vi "peak_detection.vi"(9 "spectrum cluster":T1, 10 "Minimum Peak Width":i32=5 min=3, 11 "Threshold Value":dbl=10.0) -> (1 "PeaksFound":i32)   [LabVIEW 2012]
uses:
  <vilib>/Analysis/baseanly.llb/Mean (DBL).vi
  <vilib>/measure/NI_MAPro.lvlib
  <vilib>/Analysis/NI_AALBase.lvlib
panel:
  in  "Stop":bool
  out "Amplitude":dbl[](array[numeric]) format="%.3p"
  out "Frequency":dbl[](array[numeric]) format="%.6p"
  out "Average Cor":cluster{"Array":dbl[], "magnitude":dbl[]}[](graph)
  # "Peak Detection"
  # "Detection Settings"
  # "Detected Peaks"
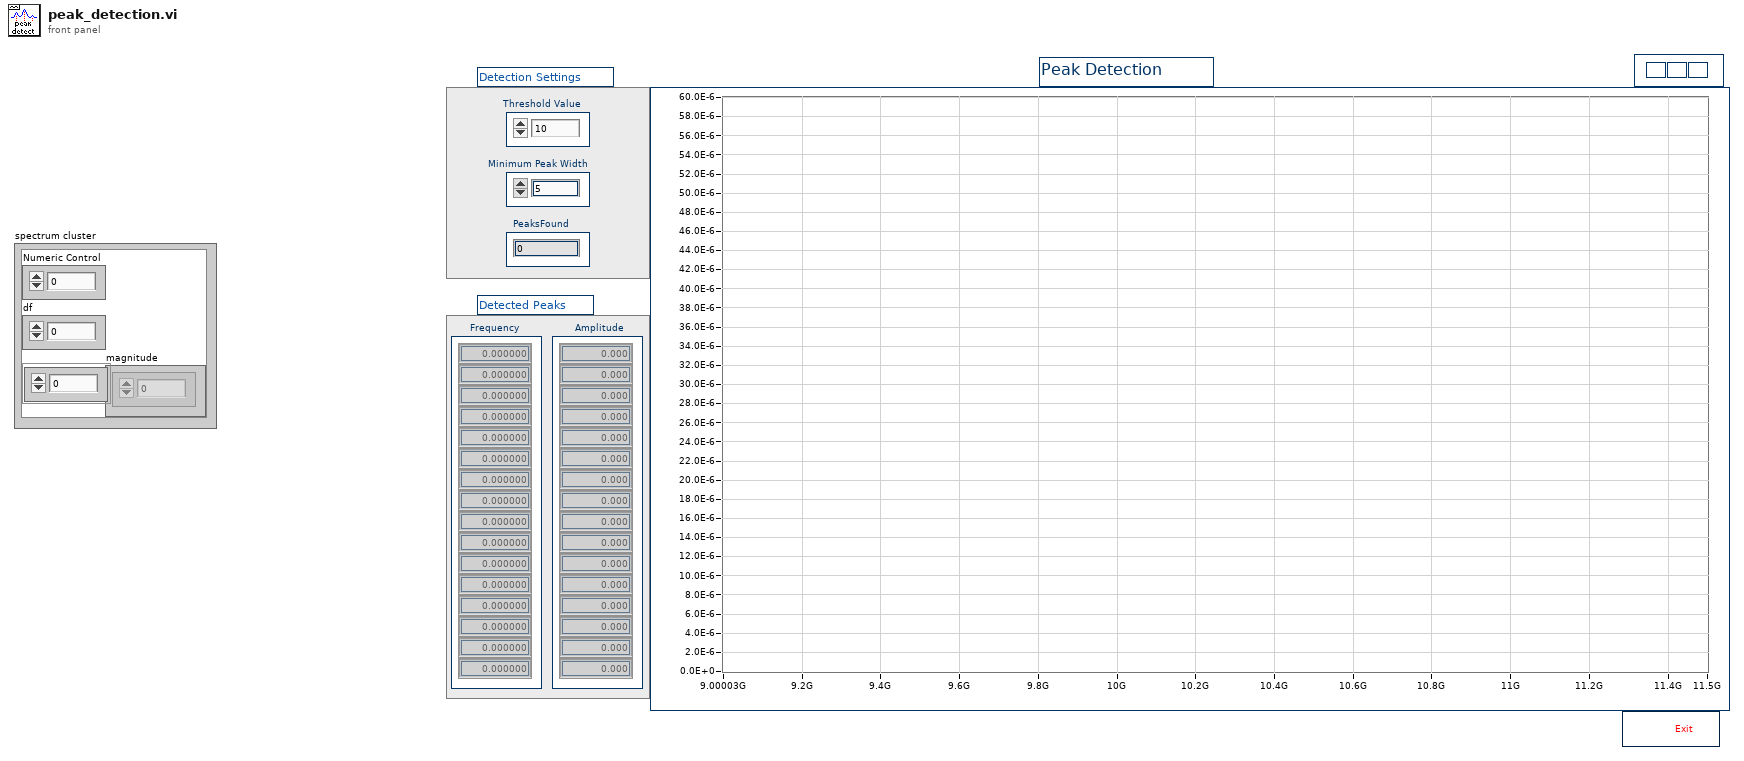
[diagram p1: front panel]
types:
  T1 = cluster{"Numeric Control":dbl, "df":dbl, "magnitude":dbl[]}
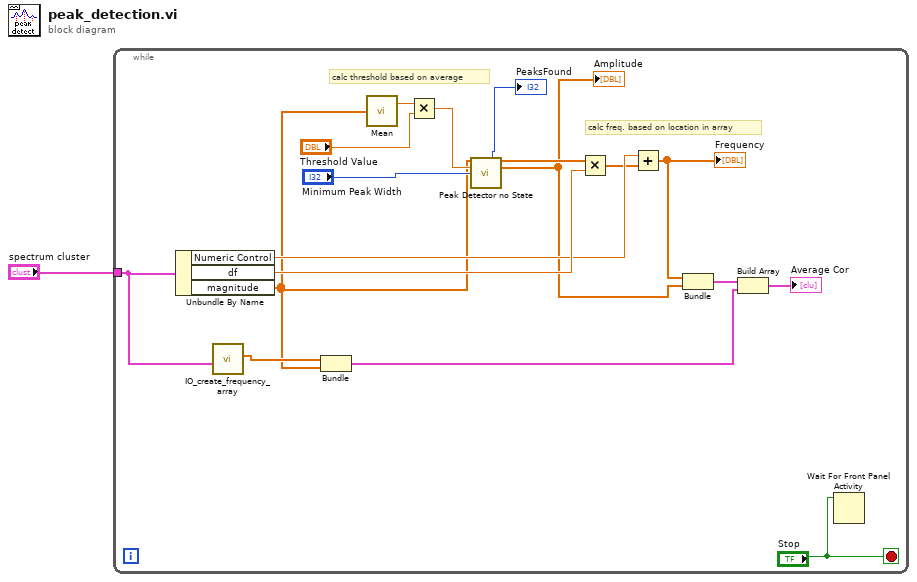
[diagram p0: block diagram]
diagram:
  n1 = while {
    tunnel: "spectrum cluster" -> [w5]
    stop <- "Stop" stop-if-true
    # "calc freq. based on location in array"
    # "calc threshold based on average"
    n2 = Unbundle By Name(w5) -> ("Numeric Control"=w13:dbl, "df"=w14:dbl, "magnitude"=w9:dbl[])
    n3 = call "IO_create_frequency_array.vi"("cor"=w5) -> ("Array"=w10:dbl[])  [unwired: 9 in, 1 out]
    n4 = Bundle("Array"=w10, "magnitude"=w9) -> (w6:cluster{"Array":dbl[], "magnitude":dbl[]})  [unwired: 1 in]
    n5 = call-poly <vilib>:"Mean.vi"("X"=w9) -> ("mean"=w17:dbl)  [unwired: 1 out]
    n6 = Multiply(x=w17, y="Threshold Value") -> (x*y=w11:dbl)
    n7 = call <vilib>:"Peak Detector no State.vi"("X"=w9, "threshold"=w11, "width"="Minimum Peak Width") -> ("# found"=→"PeaksFound":i32, "Locations"=w15:dbl[], "Amplitudes"=w3:dbl[])  [unwired: 5 in, 5 out]
    "Amplitude" <- w3
    n8 = Multiply(x=w15, y=w14) -> (x*y=w12:dbl[])
    n9 = Add(x=w13, y=w12) -> (x+y=w8:dbl[])
    "Frequency" <- w8
    n10 = Bundle(w8, "Amplitudes"=w3) -> (w7:cluster{dbl[], "Amplitudes":dbl[]})  [unwired: 1 in]
    n11 = Build Array(w7, w6) -> (→"Average Cor":cluster{"Array":dbl[], "magnitude":dbl[]}[])
    n12 = Wait For Front Panel Activity(3:"Stop") -> ()  [unwired: 2 in, 1 out]
  }
